vi "mbtest.vi"() -> ()   [LabVIEW 2015]
uses:
  libraries/ModBUS.lvlibp/ASCII/ASCII.lvclass
panel:
  out "string":string
  out "Data":i16[](array[numeric])
  out "Finished":bool
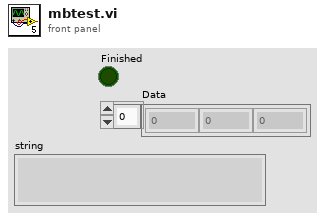
[diagram p1: front panel]
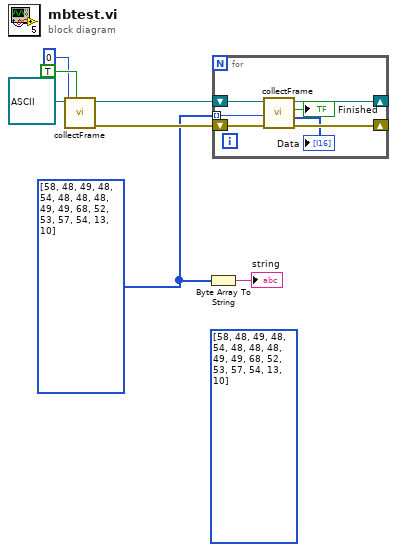
[diagram p0: block diagram]
diagram:
  (unwired) u8[] [58, 48, 49, 48, 54, 48, 48, 48, 49, 49, 68, 52, 53, 57, 54, 13, 10]
  w2 = u8[] [58, 48, 49, 48, 54, 48, 48, 48, 49, 49, 68, 52, 53, 57, 54, 13, 10]
  n1 = call-dynamic "collectFrame.vi"("Reset"=TRUE, "byte"=u8 0, "ASCII in"=refnum<class "ASCII.lvclass"> refnum) -> ("error out"=w7:errorcluster, "ASCII out"=w6:refnum<class "ASCII.lvclass">)  [unwired: 4 in, 3 out]
  n2 = Byte Array To String(unsigned byte array=w2) -> (string=→"string":string)
  n3 = for {
    shift-right: [w13] -> _
    shift-left: w7 -> [w14]
    shift-right: [w11] -> _
    shift-left: w6 -> [w12]
    tunnel: w2 -> [w10] mode=indexing
    n4 = call-dynamic "collectFrame.vi"("error in (no error)"=w14, "byte"=w10, "ASCII in"=w12) -> ("error out"=w13:errorcluster, "Data"=→"Data":i16[], "Finished"=→"Finished":bool, "ASCII out"=w11:refnum<class "ASCII.lvclass">)  [unwired: 4 in, 1 out]
  }
